vi "FM_RTL-SDR_RX_atan2_DLL_X64.vi"() -> (3 "Calculation Time (s)":dbl)   [LabVIEW 2013]
doc: "Demonstrates how to use the MATLAB script node. The m-file script is used to calculate the data and the resulting fractal is displayed on the front panel. The MathWorks, Inc. MATLAB (R) Application Software version 5.0 or later must be installed and properly licensed in order to run this VI."
uses:
  <vilib>/Waveform/WDTFileIO.llb/Read Waveform from File.vi
  <userlib>/FMDemodRTLSDR_Script/FMDemodRTLSDR_Script.dll
panel:
  out "error out":errorcluster
  in  "error in (no error)":errorcluster
  out "Baseband":dbl[](array[numeric])
  in  "file path":path=path "D:/File/Recoder_Data_IQIQ"
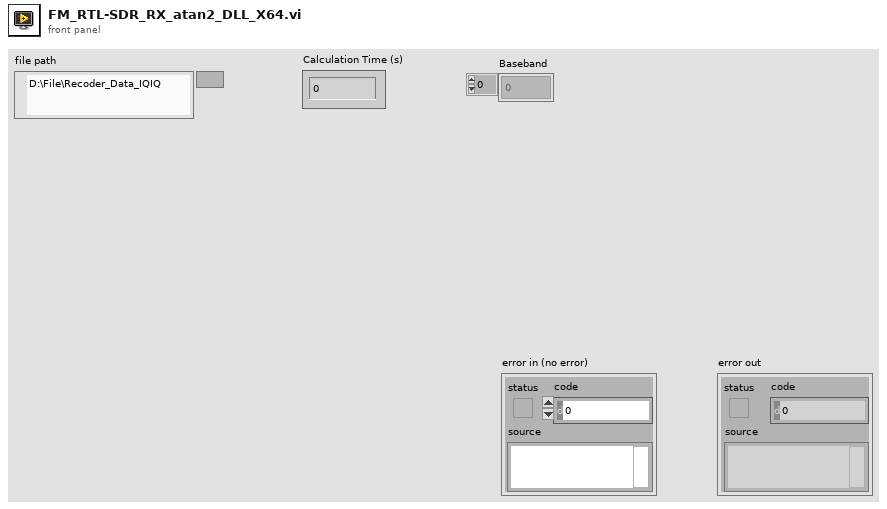
[diagram p1: front panel]
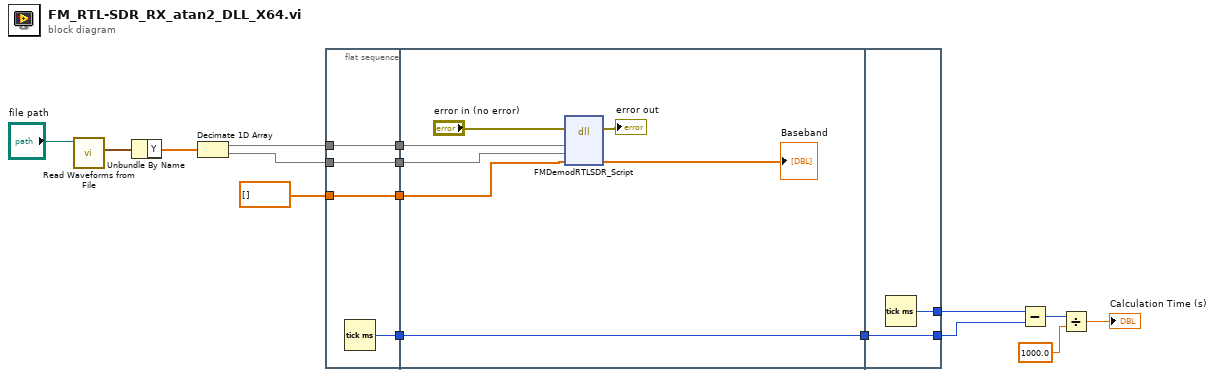
[diagram p0: block diagram]
diagram:
  n1 = call-poly <vilib>:"Read Waveforms from File.vi"("file path (dialog if empty)"="file path") -> ("first waveform in record"=w9:waveform(dbl))  [unwired: 5 in, 3 out]
  n2 = Unbundle By Name(w9) -> ("Y"=w7:dbl[])
  n3 = Decimate 1D Array(w7) -> (w5:dbl[], w3:dbl[])
  n4 = flat-sequence {
    tunnel: [w20] -> w10
    tunnel: [w19] -> w6
    tunnel: w5 -> [w19]
    tunnel: [w18] -> w4
    tunnel: w3 -> [w18]
    tunnel: dbl[] [] ("Phase_Diff") -> [w17]
    tunnel: [w17] -> w1
    tunnel: [w27] -> w16
    tunnel: w10 -> [w27]
    tunnel: w6 -> [w23]
    tunnel: w4 -> [w22]
    tunnel: w1 -> [w21]
    tunnel: w16 -> [w28]
    tunnel: [w29] -> w13
    tunnel: [w28] -> w12
    frame #0 {
      n5 = Tick Count (ms)() -> (millisecond timer value=w20:u32)
    }
    frame #1 {
      n6 = dll-call lib="C:/Program Files/National Instruments/LabVIEW 2013/user.lib/FMDemodRTLSDR_Script/FMDemodRTLSDR_Script.*" fn="FMDemodRTLSDR_Script"(error in="error in (no error)", "ISamples"=w23, "QSamples"=w22, "Phase_Diff"=w21) -> (error out=→"error out":errorcluster, "Phase_Diff"=→"Baseband":dbl[])  [unwired: 5 in, 1 out]
    }
    frame #2 {
      n7 = Tick Count (ms)() -> (millisecond timer value=w29:u32)
    }
  }
  n8 = Subtract(x=w13, y=w12) -> (x-y=w14:u32)
  n9 = Divide(x=w14, y=1000.0) -> (x/y=→"Calculation Time (s)":dbl)
